vi "test TCX read (installed 71).vi"() -> ()   [LabVIEW 2011] (continued)
ts></TPX></Extensions></Trackpoint><Trackpoint><Time>2008-03-03T14:03:14Z</Time><Position><LatitudeDegrees>35.862978</LatitudeDegrees><LongitudeDegrees>-78.901660</LongitudeDegrees></Position><AltitudeMeters>94.827</AltitudeMeters><DistanceMeters>7936.581</DistanceMeters><Cadence>76</Cadence><Extensions><TPX xmlns=\"http://www.garmin.com/xmlschemas/ActivityExtension/v2\"><Watts>189</Watts></TPX></Extensions></Trackpoint><Trackpoint><Time>2008-03-03T14:03:15Z</Time><Position><LatitudeDegrees>35.862989</LatitudeDegrees><LongitudeDegrees>-78.901582</LongitudeDegrees></Position><AltitudeMeters>94.347</AltitudeMeters><DistanceMeters>7943.796</DistanceMeters><Cadence>76</Cadence><Extensions><TPX xmlns=\"http://www.garmin.com/xmlschemas/ActivityExtension/v2\"><Watts>189</Watts></TPX></Extensions></Trackpoint><Trackpoint><Time>2008-03-03T14:03:16Z</Time><Position><LatitudeDegrees>35.863009</LatitudeDegrees><LongitudeDegrees>-78.901503</LongitudeDegrees></Position><AltitudeMeters>94.347</AltitudeMeters><DistanceMeters>7951.251</DistanceMeters><Cadence>78</Cadence><Extensions><TPX xmlns=\"http://www.garmin.com/xmlschemas/ActivityExtension/v2\"><Watts>185</Watts></TPX></Extensions></Trackpoint><Trackpoint><Time>2008-03-03T14:03:17Z</Time><Position><LatitudeDegrees>35.863023</LatitudeDegrees><LongitudeDegrees>-78.901423</LongitudeDegrees></Position><AltitudeMeters>94.347</AltitudeMeters><DistanceMeters>7958.711</DistanceMeters><Cadence>78</Cadence><Extensions><TPX xmlns=\"http://www.garmin.com/xmlschemas/ActivityExtension/v2\"><Watts>184</Watts></TPX></Extensions></Trackpoint><Trackpoint><Time>2008-03-03T14:03:18Z</Time><Position><LatitudeDegrees>35.863042</LatitudeDegrees><LongitudeDegrees>-78.901342</LongitudeDegrees></Position><AltitudeMeters>94.347</AltitudeMeters><DistanceMeters>7966.281</DistanceMeters><Cadence>72</Cadence><Extensions><TPX xmlns=\"http://www.garmin.com/xmlschemas/ActivityExtension/v2\"><Watts>157</Watts></TPX></Extensions></Trackpoint><Trackpoint><Time>2008-03-03T14:03:19Z</Time><Position><LatitudeDegrees>35.863061</LatitudeDegrees><LongitudeDegrees>-78.901258</LongitudeDegrees></Position><AltitudeMeters>94.347</AltitudeMeters><DistanceMeters>7974.119</DistanceMeters><Cadence>73</Cadence><Extensions><TPX xmlns=\"http://www.garmin.com/xmlschemas/ActivityExtension/v2\"><Watts>157</Watts></TPX></Extensions></Trackpoint><Trackpoint><Time>2008-03-03T14:03:20Z</Time><Position><LatitudeDegrees>35.863074</LatitudeDegrees><LongitudeDegrees>-78.901173</LongitudeDegrees></Position><AltitudeMeters>94.347</AltitudeMeters><DistanceMeters>7981.873</DistanceMeters><Cadence>73</Cadence><Extensions><TPX xmlns=\"http://www.garmin.com/xmlschemas/ActivityExtension/v2\"><Watts>156</Watts></TPX></Extensions></Trackpoint><Trackpoint><Time>2008-03-03T14:03:21Z</Time><Position><LatitudeDegrees>35.863089</LatitudeDegrees><LongitudeDegrees>-78.901086</LongitudeDegrees></Position><AltitudeMeters>94.347</AltitudeMeters><DistanceMeters>7989.980</DistanceMeters><Cadence>78</Cadence><Extensions><TPX xmlns=\"http://www.garmin.com/xmlschemas/ActivityExtension/v2\"><Watts>181</Watts></TPX></Extensions></Trackpoint><Trackpoint><Time>2008-03-03T14:03:22Z</Time><Position><LatitudeDegrees>35.863110</LatitudeDegrees><LongitudeDegrees>-78.900992</LongitudeDegrees></Position><AltitudeMeters>93.866</AltitudeMeters><DistanceMeters>7998.730</DistanceMeters><Cadence>80</Cadence><Extensions><TPX xmlns=\"http://www.garmin.com/xmlschemas/ActivityExtension/v2\"><Watts>180</Watts></TPX></Extensions></Trackpoint><Trackpoint><Time>2008-03-03T14:03:23Z</Time><Position><LatitudeDegrees>35.863126</LatitudeDegrees><LongitudeDegrees>-78.900894</LongitudeDegrees></Position><AltitudeMeters>93.866</AltitudeMeters><DistanceMeters>8007.869</DistanceMeters><Cadence>83</Cadence><Extensions><TPX xmlns=\"http://www.garmin.com/xmlschemas/ActivityExtension/v2\"><Watts>159</Watts></TPX></Extensions></Trackpoint><Trackpoint><Time>2008-03-03T14:03:24Z</Time><Position><LatitudeDegrees>35.863147</LatitudeDegrees><LongitudeDegrees>-78.900793</LongitudeDegrees></Position><AltitudeMeters>93.866</AltitudeMeters><DistanceMeters>8017.229</DistanceMeters><Cadence>88</Cadence><Extensions><TPX xmlns=\"http://www.garmin.com/xmlschemas/ActivityExtension/v2\"><Watts>159</Watts></TPX></Extensions></Trackpoint><Trackpoint><Time>2008-03-03T14:03:25Z</Time><Position><LatitudeDegrees>35.863168</LatitudeDegrees><LongitudeDegrees>-78.900690</LongitudeDegrees></Position><AltitudeMeters>93.385</AltitudeMeters><DistanceMeters>8026.872</DistanceMeters><Cadence>88</Cadence><Extensions><TPX xmlns=\"http://www.garmin.com/xmlschemas/ActivityExtension/v2\"><Watts>159</Watts></TPX></Extensions></Trackpoint><Trackpoint><Time>2008-03-03T14:03:26Z</Time><Position><LatitudeDegrees>35.863186</LatitudeDegrees><LongitudeDegrees>-78.900583</LongitudeDegrees></Position><AltitudeMeters>92.905</AltitudeMeters><DistanceMeters>8036.698</DistanceMeters><Cadence>91</Cadence><Extensions><TPX xmlns=\"http://www.garmin.com/xmlschemas/ActivityExtension/v2\"><Watts>143</Watts></TPX></Extensions></Trackpoint><Trackpoint><Time>2008-03-03T14:03:27Z</Time><Position><LatitudeDegrees>35.863206</LatitudeDegrees><LongitudeDegrees>-78.900473</LongitudeDegrees></Position><AltitudeMeters>92.905</AltitudeMeters><DistanceMeters>8046.873</DistanceMeters><Cadence>91</Cadence><Extensions><TPX xmlns=\"http://www.garmin.com/xmlschemas/ActivityExtension/v2\"><Watts>142</Watts></TPX></Extensions></Trackpoint><Trackpoint><Time>2008-03-03T14:03:28Z</Time><Position><LatitudeDegrees>35.863225</LatitudeDegrees><LongitudeDegrees>-78.900361</LongitudeDegrees></Position><AltitudeMeters>92.424</AltitudeMeters><DistanceMeters>8057.292</DistanceMeters><Cadence>91</Cadence><Extensions><TPX xmlns=\"http://www.garmin.com/xmlschemas/ActivityExtension/v2\"><Watts>149</Watts></TPX></Extensions></Trackpoint><Trackpoint><Time>2008-03-03T14:03:29Z</Time><Position><LatitudeDegrees>35.863246</LatitudeDegrees><LongitudeDegrees>-78.900251</LongitudeDegrees></Position><AltitudeMeters>92.424</AltitudeMeters><DistanceMeters>8067.389</DistanceMeters><Cadence>91</Cadence><Extensions><TPX xmlns=\"http://www.garmin.com/xmlschemas/ActivityExtension/v2\"><Watts>148</Watts></TPX></Extensions></Trackpoint><Trackpoint><Time>2008-03-03T14:03:30Z</Time><Position><LatitudeDegrees>35.863261</LatitudeDegrees><LongitudeDegrees>-78.900148</LongitudeDegrees></Position><AltitudeMeters>92.905</AltitudeMeters><DistanceMeters>8076.814</DistanceMeters><Cadence>88</Cadence><Extensions><TPX xmlns=\"http://www.garmin.com/xmlschemas/ActivityExtension/v2\"><Watts>154</Watts></TPX></Extensions></Trackpoint><Trackpoint><Time>2008-03-03T14:03:31Z</Time><Position><LatitudeDegrees>35.863276</LatitudeDegrees><LongitudeDegrees>-78.900048</LongitudeDegrees></Position><AltitudeMeters>92.905</AltitudeMeters><DistanceMeters>8085.958</DistanceMeters><Cadence>84</Cadence><Extensions><TPX xmlns=\"http://www.garmin.com/xmlschemas/ActivityExtension/v2\"><Watts>164</Watts></TPX></Extensions></Trackpoint><Trackpoint><Time>2008-03-03T14:03:32Z</Time><Position><LatitudeDegrees>35.863288</LatitudeDegrees><LongitudeDegrees>-78.899952</LongitudeDegrees></Position><AltitudeMeters>92.905</AltitudeMeters><DistanceMeters>8094.699</DistanceMeters><Cadence>83</Cadence><Extensions><TPX xmlns=\"http://www.garmin.com/xmlschemas/ActivityExtension/v2\"><Watts>165</Watts></TPX></Extensions></Trackpoint><Trackpoint><Time>2008-03-03T14:03:33Z</Time><Position><LatitudeDegrees>35.863300</LatitudeDegrees><LongitudeDegrees>-78.899857</LongitudeDegrees></Position><AltitudeMeters>93.385</AltitudeMeters><DistanceMeters>8103.383</DistanceMeters><Cadence>79</Cadence><Extensions><TPX xmlns=\"http://www.garmin.com/xmlschemas/ActivityExtension/v2\"><Watts>173</Watts></TPX></Extensions></Trackpoint><Trackpoint><Time>2008-03-03T14:03:34Z</Time><Position><LatitudeDegrees>35.863310</LatitudeDegrees><LongitudeDegrees>-78.899768</LongitudeDegrees></Position><AltitudeMeters>93.385</AltitudeMeters><DistanceMeters>8111.526</DistanceMeters><Cadence>74</Cadence><Extensions><TPX xmlns=\"http://www.garmin.com/xmlschemas/ActivityExtension/v2\"><Watts>185</Watts></TPX></Extensions></Trackpoint><Trackpoint><Time>2008-03-03T14:03:35Z</Time><Position><LatitudeDegrees>35.863325</LatitudeDegrees><LongitudeDegrees>-78.899681</LongitudeDegrees></Position><AltitudeMeters>93.866</AltitudeMeters><DistanceMeters>8119.541</DistanceMeters><Cadence>74</Cadence><Extensions><TPX xmlns=\"http://www.garmin.com/xmlschemas/ActivityExtension/v2\"><Watts>186</Watts></TPX></Extensions></Trackpoint><Trackpoint><Time>2008-03-03T14:03:36Z</Time><Position><LatitudeDegrees>35.863345</LatitudeDegrees><LongitudeDegrees>-78.899593</LongitudeDegrees></Position><AltitudeMeters>93.866</AltitudeMeters><DistanceMeters>8127.668</DistanceMeters><Cadence>75</Cadence><Extensions><TPX xmlns=\"http://www.garmin.com/xmlschemas/ActivityExtension/v2\"><Watts>416</Watts></TPX></Extensions></Trackpoint><Trackpoint><Time>2008-03-03T14:03:37Z</Time><Position><LatitudeDegrees>35.863368</LatitudeDegrees><LongitudeDegrees>-78.899510</LongitudeDegrees></Position><AltitudeMeters>94.827</AltitudeMeters><DistanceMeters>8135.531</DistanceMeters><Cadence>75</Cadence><Extensions><TPX xmlns=\"http://www.garmin.com/xmlschemas/ActivityExtension/v2\"><Watts>415</Watts></TPX></Extensions></Trackpoint><Trackpoint><Time>2008-03-03T14:03:38Z</Time><Position><LatitudeDegrees>35.863381</LatitudeDegrees><LongitudeDegrees>-78.899422</LongitudeDegrees></Position><AltitudeMeters>94.827</AltitudeMeters><DistanceMeters>8143.633</DistanceMeters><Cadence>77</Cadence><Extensions><TPX xmlns=\"http://www.garmin.com/xmlschemas/ActivityExtension/v2\"><Watts>685</Watts></TPX></Extensions></Trackpoint><Trackpoint><Time>2008-03-03T14:03:39Z</Time><Position><LatitudeDegrees>35.863397</LatitudeDegrees><LongitudeDegrees>-78.899329</LongitudeDegrees></Position><AltitudeMeters>95.308</AltitudeMeters><DistanceMeters>8152.224</DistanceMeters><Cadence>78</Cadence><Extensions><TPX xmlns=\"http://www.garmin.com/xmlschemas/ActivityExtension/v2\"><Watts>675</Watts></TPX></Extensions></Trackpoint><Trackpoint><Time>2008-03-03T14:03:40Z</Time><Position><LatitudeDegrees>35.863421</LatitudeDegrees><LongitudeDegrees>-78.899235</LongitudeDegrees></Position><AltitudeMeters>95.788</AltitudeMeters><DistanceMeters>8161.086</DistanceMeters><Cadence>79</Cadence><Extensions><TPX xmlns=\"http://www.garmin.com/xmlschemas/ActivityExtension/v2\"><Watts>674</Watts></TPX></Extensions></Trackpoint><Trackpoint><Time>2008-03-03T14:03:41Z</Time><Position><LatitudeDegrees>35.863439</LatitudeDegrees><LongitudeDegrees>-78.899142</LongitudeDegrees></Position><AltitudeMeters>96.269</AltitudeMeters><DistanceMeters>8169.801</DistanceMeters><Cadence>79</Cadence><Extensions><TPX xmlns=\"http://www.garmin.com/xmlschemas/ActivityExtension/v2\"><Watts>667</Watts></TPX></Extensions></Trackpoint><Trackpoint><Time>2008-03-03T14:03:42Z</Time><Position><LatitudeDegrees>35.863455</LatitudeDegrees><LongitudeDegrees>-78.899045</LongitudeDegrees></Position><AltitudeMeters>96.269</AltitudeMeters><DistanceMeters>8178.699</DistanceMeters><Cadence>79</Cadence><Extensions><TPX xmlns=\"http://www.garmin.com/xmlschemas/ActivityExtension/v2\"><Watts>670</Watts></TPX></Extensions></Trackpoint><Trackpoint><Time>2008-03-03T14:03:43Z</Time><Position><LatitudeDegrees>35.863473</LatitudeDegrees><LongitudeDegrees>-78.898952</LongitudeDegrees></Position><AltitudeMeters>96.750</AltitudeMeters><DistanceMeters>8187.334</DistanceMeters><Cadence>79</Cadence><Extensions><TPX xmlns=\"http://www.garmin.com/xmlschemas/ActivityExtension/v2\"><Watts>540</Watts></TPX></Extensions></Trackpoint><Trackpoint><Time>2008-03-03T14:03:44Z</Time><Position><LatitudeDegrees>35.863492</LatitudeDegrees><LongitudeDegrees>-78.898856</LongitudeDegrees></Position><AltitudeMeters>96.750</AltitudeMeters><DistanceMeters>8196.224</DistanceMeters><Cadence>79</Cadence><Extensions><TPX xmlns=\"http://www.garmin.com/xmlschemas/ActivityExtension/v2\"><Watts>544</Watts></TPX></Extensions></Trackpoint><Trackpoint><Time>2008-03-03T14:03:45Z</Time><Position><LatitudeDegrees>35.863502</LatitudeDegrees><LongitudeDegrees>-78.898763</LongitudeDegrees></Position><AltitudeMeters>97.711</AltitudeMeters><DistanceMeters>8204.663</DistanceMeters><Cadence>79</Cadence><Extensions><TPX xmlns=\"http://www.garmin.com/xmlschemas/ActivityExtension/v2\"><Watts>541</Watts></TPX></Extensions></Trackpoint><Trackpoint><Time>2008-03-03T14:03:46Z</Time><Position><LatitudeDegrees>35.863514</LatitudeDegrees><LongitudeDegrees>-78.898672</LongitudeDegrees></Position><AltitudeMeters>97.711</AltitudeMeters><DistanceMeters>8212.996</DistanceMeters><Cadence>78</Cadence><Extensions><TPX xmlns=\"http://www.garmin.com/xmlschemas/ActivityExtension/v2\"><Watts>515</Watts></TPX></Extensions></Trackpoint><Trackpoint><Time>2008-03-03T14:03:47Z</Time><Position><LatitudeDegrees>35.863528</LatitudeDegrees><LongitudeDegrees>-78.898578</LongitudeDegrees></Position><AltitudeMeters>98.192</AltitudeMeters><DistanceMeters>8221.674</DistanceMeters><Cadence>79</Cadence><Extensions><TPX xmlns=\"http://www.garmin.com/xmlschemas/ActivityExtension/v2\"><Watts>507</Watts></TPX></Extensions></Trackpoint><Trackpoint><Time>2008-03-03T14:03:48Z</Time><Position><LatitudeDegrees>35.863539</LatitudeDegrees><LongitudeDegrees>-78.898486</LongitudeDegrees></Position><AltitudeMeters>98.192</AltitudeMeters><DistanceMeters>8230.088</DistanceMeters><Cadence>79</Cadence><Extensions><TPX xmlns=\"http://www.garmin.com/xmlschemas/ActivityExtension/v2\"><Watts>482</Watts></TPX></Extensions></Trackpoint><Trackpoint><Time>2008-03-03T14:03:49Z</Time><Position><LatitudeDegrees>35.863548</LatitudeDegrees><LongitudeDegrees>-78.898391</LongitudeDegrees></Position><AltitudeMeters>99.153</AltitudeMeters><DistanceMeters>8238.679</DistanceMeters><Cadence>81</Cadence><Extensions><TPX xmlns=\"http://www.garmin.com/xmlschemas/ActivityExtension/v2\"><Watts>470</Watts></TPX></Extensions></Trackpoint><Trackpoint><Time>2008-03-03T14:03:50Z</Time><Position><LatitudeDegrees>35.863565</LatitudeDegrees><LongitudeDegrees>-78.898296</LongitudeDegrees></Position><AltitudeMeters>99.153</AltitudeMeters><DistanceMeters>8247.451</DistanceMeters><Cadence>78</Cadence><Extensions><TPX xmlns=\"http://www.garmin.com/xmlschemas/ActivityExtension/v2\"><Watts>381</Watts></TPX></Extensions></Trackpoint><Trackpoint><Time>2008-03-03T14:03:51Z</Time><Position><LatitudeDegrees>35.863576</LatitudeDegrees><LongitudeDegrees>-78.898206</LongitudeDegrees></Position><AltitudeMeters>99.634</AltitudeMeters><DistanceMeters>8255.699</DistanceMeters><Cadence>77</Cadence><Extensions><TPX xmlns=\"http://www.garmin.com/xmlschemas/ActivityExtension/v2\"><Watts>278</Watts></TPX></Extensions></Trackpoint><Trackpoint><Time>2008-03-03T14:03:52Z</Time><Position><LatitudeDegrees>35.863592</LatitudeDegrees><LongitudeDegrees>-78.898116</LongitudeDegrees></Position><AltitudeMeters>99.634</AltitudeMeters><DistanceMeters>8264.034</DistanceMeters><Cadence>77</Cadence><Extensions><TPX xmlns=\"http://www.garmin.com/xmlschemas/ActivityExtension/v2\"><Watts>278</Watts></TPX></Extensions></Trackpoint><Trackpoint><Time>2008-03-03T14:03:53Z</Time><Position><LatitudeDegrees>35.863607</LatitudeDegrees><LongitudeDegrees>-78.898024</LongitudeDegrees></Position><AltitudeMeters>100.115</AltitudeMeters><DistanceMeters>8272.420</DistanceMeters><Cadence>75</Cadence><Extensions><TPX xmlns=\"http://www.garmin.com/xmlschemas/ActivityExtension/v2\"><Watts>223</Watts></TPX></Extensions></Trackpoint><Trackpoint><Time>2008-03-03T14:03:54Z</Time><Position><LatitudeDegrees>35.863619</LatitudeDegrees><LongitudeDegrees>-78.897934</LongitudeDegrees></Position><AltitudeMeters>100.115</AltitudeMeters><DistanceMeters>8280.670</DistanceMeters><Cadence>75</Cadence><Extensions><TPX xmlns=\"http://www.garmin.com/xmlschemas/ActivityExtension/v2\"><Watts>222</Watts></TPX></Extensions></Trackpoint><Trackpoint><Time>2008-03-03T14:03:55Z</Time><Position><LatitudeDegrees>35.863635</LatitudeDegrees><LongitudeDegrees>-78.897846</LongitudeDegrees></Position><AltitudeMeters>100.115</AltitudeMeters><DistanceMeters>8288.826</DistanceMeters><Cadence>73</Cadence><Extensions><TPX xmlns=\"http://www.garmin.com/xmlschemas/ActivityExtension/v2\"><Watts>224</Watts></TPX></Extensions></Trackpoint><Trackpoint><Time>2008-03-03T14:03:56Z</Time><Position><LatitudeDegrees>35.863646</LatitudeDegrees><LongitudeDegrees>-78.897761</LongitudeDegrees></Position><AltitudeMeters>100.115</AltitudeMeters><DistanceMeters>8296.627</DistanceMeters><Cadence>73</Cadence><Extensions><TPX xmlns=\"http://www.garmin.com/xmlschemas/ActivityExtension/v2\"><Watts>224</Watts></TPX></Extensions></Trackpoint><Trackpoint><Time>2008-03-03T14:03:57Z</Time><Position><LatitudeDegrees>35.863663</LatitudeDegrees><LongitudeDegrees>-78.897678</LongitudeDegrees></Position><AltitudeMeters>100.595</AltitudeMeters><DistanceMeters>8304.372</DistanceMeters><Cadence>72</Cadence><Extensions><TPX xmlns=\"http://www.garmin.com/xmlschemas/ActivityExtension/v2\"><Watts>221</Watts></TPX></Extensions></Trackpoint><Trackpoint><Time>2008-03-03T14:03:58Z</Time><Position><LatitudeDegrees>35.863680</LatitudeDegrees><LongitudeDegrees>-78.897595</LongitudeDegrees></Position><AltitudeMeters>100.595</AltitudeMeters><DistanceMeters>8312.060</DistanceMeters><Cadence>70</Cadence><Extensions><TPX xmlns=\"http://www.garmin.com/xmlschemas/ActivityExtension/v2\"><Watts>207</Watts></TPX></Extensions></Trackpoint><Trackpoint><Time>2008-03-03T14:03:59Z</Time><Position><LatitudeDegrees>35.863703</LatitudeDegrees><LongitudeDegrees>-78.897514</LongitudeDegrees></Position><AltitudeMeters>101.076</AltitudeMeters><DistanceMeters>8319.789</DistanceMeters><Cadence>69</Cadence><Extensions><TPX xmlns=\"http://www.garmin.com/xmlschemas/ActivityExtension/v2\"><Watts>193</Watts></TPX></Extensions></Trackpoint><Trackpoint><Time>2008-03-03T14:04:00Z</Time><Position><LatitudeDegrees>35.863717</LatitudeDegrees><LongitudeDegrees>-78.897436</LongitudeDegrees></Position><AltitudeMeters>101.076</AltitudeMeters><DistanceMeters>8327.021</DistanceMeters><Cadence>67</Cadence><Extensions><TPX xmlns=\"http://www.garmin.com/xmlschemas/ActivityExtension/v2\"><Watts>198</Watts></TPX></Extensions></Trackpoint><Trackpoint><Time>2008-03-03T14:04:01Z</Time><Position><LatitudeDegrees>35.863723</LatitudeDegrees><LongitudeDegrees>-78.897357</LongitudeDegrees></Position><AltitudeMeters>101.076</AltitudeMeters><DistanceMeters>8334.132</DistanceMeters><Cadence>67</Cadence><Extensions><TPX xmlns=\"http://www.garmin.com/xmlschemas/ActivityExtension/v2\"><Watts>215</Watts></TPX></Extensions></Trackpoint><Trackpoint><Time>2008-03-03T14:04:02Z</Time><Position><LatitudeDegrees>35.863730</LatitudeDegrees><LongitudeDegrees>-78.897280</LongitudeDegrees></Position><AltitudeMeters>101.076</AltitudeMeters><DistanceMeters>8341.184</DistanceMeters><Cadence>67</Cadence><Extensions><TPX xmlns=\"http://www.garmin.com/xmlschemas/ActivityExtension/v2\"><Watts>213</Watts></TPX></Extensions></Trackpoint><Trackpoint><Time>2008-03-03T14:04:03Z</Time><Position><LatitudeDegrees>35.863739</LatitudeDegrees><LongitudeDegrees>-78.897199</LongitudeDegrees></Position><AltitudeMeters>101.076</AltitudeMeters><DistanceMeters>8348.546</DistanceMeters><Cadence>67</Cadence><Extensions><TPX xmlns=\"http://www.garmin.com/xmlschemas/ActivityExtension/v2\"><Watts>230</Watts></TPX></Extensions></Trackpoint><Trackpoint><Time>2008-03-03T14:04:04Z</Time><Position><LatitudeDegrees>35.863747</LatitudeDegrees><LongitudeDegrees>-78.897118</LongitudeDegrees></Position><AltitudeMeters>101.076</AltitudeMeters><DistanceMeters>8355.904</DistanceMeters><Cadence>67</Cadence><Extensions><TPX xmlns=\"http://www.garmin.com/xmlschemas/ActivityExtension/v2\"><Watts>232</Watts></TPX></Extensions></Trackpoint><Trackpoint><Time>2008-03-03T14:04:05Z</Time><Position><LatitudeDegrees>35.863738</LatitudeDegrees><LongitudeDegrees>-78.897041</LongitudeDegrees></Position><AltitudeMeters>101.076</AltitudeMeters><DistanceMeters>8362.927</DistanceMeters><Cadence>66</Cadence><Extensions><TPX xmlns=\"http://www.garmin.com/xmlschemas/ActivityExtension/v2\"><Watts>158</Watts></TPX></Extensions></Trackpoint><Trackpoint><Time>2008-03-03T14:04:06Z</Time><Position><LatitudeDegrees>35.863710</LatitudeDegrees><LongitudeDegrees>-78.896976</LongitudeDegrees></Position><AltitudeMeters>101.556</AltitudeMeters><DistanceMeters>8369.553</DistanceMeters><Cadence>66</Cadence><Extensions><TPX xmlns=\"http://www.garmin.com/xmlschemas/ActivityExtension/v2\"><Watts>141</Watts></TPX></Extensions></Trackpoint><Trackpoint><Time>2008-03-03T14:04:07Z</Time><Position><LatitudeDegrees>35.863647</LatitudeDegrees><LongitudeDegrees>-78.896943</LongitudeDegrees></Position><AltitudeMeters>101.556</AltitudeMeters><DistanceMeters>8377.287</DistanceMeters><Cadence>66</Cadence><Extensions><TPX xmlns=\"http://www.garmin.com/xmlschemas/ActivityExtension/v2\"><Watts>141</Watts></TPX></Extensions></Trackpoint><Trackpoint><Time>2008-03-03T14:04:08Z</Time><Position><LatitudeDegrees>35.863588</LatitudeDegrees><LongitudeDegrees>-78.896935</LongitudeDegrees></Position><AltitudeMeters>101.556</AltitudeMeters><DistanceMeters>8383.846</DistanceMeters><Cadence>66</Cadence><Extensions><TPX xmlns=\"http://www.garmin.com/xmlschemas/ActivityExtension/v2\"><Watts>136</Watts></TPX></Extensions></Trackpoint><Trackpoint><Time>2008-03-03T14:04:09Z</Time><Position><LatitudeDegrees>35.863528</LatitudeDegrees><LongitudeDegrees>-78.896946</LongitudeDegrees></Position><AltitudeMeters>101.556</AltitudeMeters><DistanceMeters>8390.634</DistanceMeters><Cadence>66</Cadence><Extensions><TPX xmlns=\"http://www.garmin.com/xmlschemas/ActivityExtension/v2\"><Watts>135</Watts></TPX></Extensions></Trackpoint><Trackpoint><Time>2008-03-03T14:04:10Z</Time><Position><LatitudeDegrees>35.863467</LatitudeDegrees><LongitudeDegrees>-78.896965</LongitudeDegrees></Position><AltitudeMeters>101.556</AltitudeMeters><DistanceMeters>8397.591</DistanceMeters><Cadence>67</Cadence><Extensions><TPX xmlns=\"http://www.garmin.com/xmlschemas/ActivityExtension/v2\"><Watts>130</Watts></TPX></Extensions></Trackpoint><Trackpoint><Time>2008-03-03T14:04:11Z</Time><Position><LatitudeDegrees>35.863399</LatitudeDegrees><LongitudeDegrees>-78.896982</LongitudeDegrees></Position><AltitudeMeters>101.556</AltitudeMeters><DistanceMeters>8405.279</DistanceMeters><Cadence>67</Cadence><Extensions><TPX xmlns=\"http://www.garmin.com/xmlschemas/ActivityExtension/v2\"><Watts>141</Watts></TPX></Extensions></Trackpoint><Trackpoint><Time>2008-03-03T14:04:12Z</Time><Position><LatitudeDegrees>35.863331</LatitudeDegrees><LongitudeDegrees>-78.896996</LongitudeDegrees></Position><AltitudeMeters>101.556</AltitudeMeters><DistanceMeters>8412.914</DistanceMeters><Cadence>68</Cadence><Extensions><TPX xmlns=\"http://www.garmin.com/xmlschemas/ActivityExtension/v2\"><Watts>151</Watts></TPX></Extensions></Trackpoint><Trackpoint><Time>2008-03-03T14:04:13Z</Time><Position><LatitudeDegrees>35.863263</LatitudeDegrees><LongitudeDegrees>-78.897010</LongitudeDegrees></Position><AltitudeMeters>101.556</AltitudeMeters><DistanceMeters>8420.536</DistanceMeters><Cadence>70</Cadence><Extensions><TPX xmlns=\"http://www.garmin.com/xmlschemas/ActivityExtension/v2\"><Watts>158</Watts></TPX></Extensions></Trackpoint><Trackpoint><Time>2008-03-03T14:04:14Z</Time><Position><LatitudeDegrees>35.863190</LatitudeDegrees><LongitudeDegrees>-78.897026</LongitudeDegrees></Position><AltitudeMeters>102.037</AltitudeMeters><DistanceMeters>8428.863</DistanceMeters><Cadence>71</Cadence><Extensions><TPX xmlns=\"http://www.garmin.com/xmlschemas/ActivityExtension/v2\"><Watts>158</Watts></TPX></Extensions></Trackpoint><Trackpoint><Time>2008-03-03T14:04:15Z</Time><Position><LatitudeDegrees>35.863116</LatitudeDegrees><LongitudeDegrees>-78.897046</LongitudeDegrees></Position><AltitudeMeters>102.037</AltitudeMeters><DistanceMeters>8437.228</DistanceMeters><Cadence>72</Cadence><Extensions><TPX xmlns=\"http://www.garmin.com/xmlschemas/ActivityExtension/v2\"><Watts>132</Watts></TPX></Extensions></Trackpoint><Trackpoint><Time>2008-03-03T14:04:16Z</Time><Position><LatitudeDegrees>35.863041</LatitudeDegrees><LongitudeDegrees>-78.897060</LongitudeDegrees></Position><AltitudeMeters>102.037</AltitudeMeters><DistanceMeters>8445.677</DistanceMeters><Cadence>73</Cadence><Extensions><TPX xmlns=\"http://www.garmin.com/xmlschemas/ActivityExtension/v2\"><Watts>127</Watts></TPX></Extensions></Trackpoint><Trackpoint><Time>2008-03-03T14:04:17Z</Time><Position><LatitudeDegrees>35.862967</LatitudeDegrees><LongitudeDegrees>-78.897071</LongitudeDegrees></Position><AltitudeMeters>102.037</AltitudeMeters><DistanceMeters>8453.937</DistanceMeters><Cadence>73</Cadence><Extensions><TPX xmlns=\"http://www.garmin.com/xmlschemas/ActivityExtension/v2\"><Watts>127</Watts></TPX></Extensions></Trackpoint><Trackpoint><Time>2008-03-03T14:04:18Z</Time><Position><LatitudeDegrees>35.862899</LatitudeDegrees><LongitudeDegrees>-78.897083</LongitudeDegrees></Position><AltitudeMeters>102.037</AltitudeMeters><DistanceMeters>8461.561</DistanceMeters><Cadence>73</Cadence><Extensions><TPX xmlns=\"http://www.garmin.com/xmlschemas/ActivityExtension/v2\"><Watts>119</Watts></TPX></Extensions></Trackpoint><Trackpoint><Time>2008-03-03T14:04:19Z</Time><Position><LatitudeDegrees>35.862828</LatitudeDegrees><LongitudeDegrees>-78.897094</LongitudeDegrees></Position><AltitudeMeters>101.556</AltitudeMeters><DistanceMeters>8469.438</DistanceMeters><Cadence>73</Cadence><Extensions><TPX xmlns=\"http://www.garmin.com/xmlschemas/ActivityExtension/v2\"><Watts>120</Watts></TPX></Extensions></Trackpoint><Trackpoint><Time>2008-03-03T14:04:20Z</Time><Position><LatitudeDegrees>35.862757</LatitudeDegrees><LongitudeDegrees>-78.897104</LongitudeDegrees></Position><AltitudeMeters>101.076</AltitudeMeters><DistanceMeters>8477.459</DistanceMeters><Cadence>75</Cadence><Extensions><TPX xmlns=\"http://www.garmin.com/xmlschemas/ActivityExtension/v2\"><Watts>129</Watts></TPX></Extensions></Trackpoint><Trackpoint><Time>2008-03-03T14:04:21Z</Time><Position><LatitudeDegrees>35.862683</LatitudeDegrees><LongitudeDegrees>-78.897116</LongitudeDegrees></Position><AltitudeMeters>101.076</AltitudeMeters><DistanceMeters>8485.744</DistanceMeters><Cadence>76</Cadence><Extensions><TPX xmlns=\"http://www.garmin.com/xmlschemas/ActivityExtension/v2\"><Watts>129</Watts></TPX></Extensions></Trackpoint><Trackpoint><Time>2008-03-03T14:04:22Z</Time><Position><LatitudeDegrees>35.862610</LatitudeDegrees><LongitudeDegrees>-78.897129</LongitudeDegrees></Position><AltitudeMeters>101.076</AltitudeMeters><DistanceMeters>8493.926</DistanceMeters><Cadence>77</Cadence><Extensions><TPX xmlns=\"http://www.garmin.com/xmlschemas/ActivityExtension/v2\"><Watts>129</Watts></TPX></Extensions></Trackpoint><Trackpoint><Time>2008-03-03T14:04:23Z</Time><Position><LatitudeDegrees>35.862534</LatitudeDegrees><LongitudeDegrees>-78.897142</LongitudeDegrees></Position><AltitudeMeters>100.115</AltitudeMeters><DistanceMeters>8502.362</DistanceMeters><Cadence>78</Cadence><Extensions><TPX xmlns=\"http://www.garmin.com/xmlschemas/ActivityExtension/v2\"><Watts>116</Watts></TPX></Extensions></Trackpoint><Trackpoint><Time>2008-03-03T14:04:24Z</Time><Position><LatitudeDegrees>35.862457</LatitudeDegrees><LongitudeDegrees>-78.897159</LongitudeDegrees></Position><AltitudeMeters>100.115</AltitudeMeters><DistanceMeters>8511.070</DistanceMeters><Cadence>78</Cadence><Extensions><TPX xmlns=\"http://www.garmin.com/xmlschemas/ActivityExtension/v2\"><Watts>116</Watts></TPX></Extensions></Trackpoint><Trackpoint><Time>2008-03-03T14:04:25Z</Time><Position><LatitudeDegrees>35.862384</LatitudeDegrees><LongitudeDegrees>-78.897181</LongitudeDegrees></Position><AltitudeMeters>99.634</AltitudeMeters><DistanceMeters>8519.451</DistanceMeters><Cadence>78</Cadence><Extensions><TPX xmlns=\"http://www.garmin.com/xmlschemas/ActivityExtension/v2\"><Watts>110</Watts></TPX></Extensions></Trackpoint><Trackpoint><Time>2008-03-03T14:04:26Z</Time><Position><LatitudeDegrees>35.862311</LatitudeDegrees><LongitudeDegrees>-78.897205</LongitudeDegrees></Position><AltitudeMeters>99.153</AltitudeMeters><DistanceMeters>8527.767</DistanceMeters><Cadence>78</Cadence><Extensions><TPX xmlns=\"http://www.garmin.com/xmlschemas/ActivityExtension/v2\"><Watts>108</Watts></TPX></Extensions></Trackpoint><Trackpoint><Time>2008-03-03T14:04:27Z</Time><Position><LatitudeDegrees>35.862235</LatitudeDegrees><LongitudeDegrees>-78.897229</LongitudeDegrees></Position><AltitudeMeters>98.672</AltitudeMeters><DistanceMeters>8536.483</DistanceMeters><Cadence>80</Cadence><Extensions><TPX xmlns=\"http://www.garmin.com/xmlschemas/ActivityExtension/v2\"><Watts>104</Watts></TPX></Extensions></Trackpoint><Trackpoint><Time>2008-03-03T14:04:28Z</Time><Position><LatitudeDegrees>35.862161</LatitudeDegrees><LongitudeDegrees>-78.897257</LongitudeDegrees></Position><AltitudeMeters>99.153</AltitudeMeters><DistanceMeters>8545.181</DistanceMeters><Cadence>81</Cadence><Extensions><TPX xmlns=\"http://www.garmin.com/xmlschemas/ActivityExtension/v2\"><Watts>101</Watts></TPX></Extensions></Trackpoint><Trackpoint><Time>2008-03-03T14:04:29Z</Time><Position><LatitudeDegrees>35.862088</LatitudeDegrees><LongitudeDegrees>-78.897289</LongitudeDegrees></Position><AltitudeMeters>98.672</AltitudeMeters><DistanceMeters>8553.725</DistanceMeters><Cadence>81</Cadence><Extensions><TPX xmlns=\"http://www.garmin.com/xmlschemas/ActivityExtension/v2\"><Watts>102</Watts></TPX></Extensions></Trackpoint><Trackpoint><Time>2008-03-03T14:04:30Z</Time><Position><LatitudeDegrees>35.862015</LatitudeDegrees><LongitudeDegrees>-78.897322</LongitudeDegrees></Position><AltitudeMeters>99.153</AltitudeMeters><DistanceMeters>8562.310</DistanceMeters><Cadence>72</Cadence><Extensions><TPX xmlns=\"http://www.garmin.com/xmlschemas/ActivityExtension/v2\"><Watts>99</Watts></TPX></Extensions></Trackpoint><Trackpoint><Time>2008-03-03T14:04:31Z</Time><Position><LatitudeDegrees>35.861941</LatitudeDegrees><LongitudeDegrees>-78.897358</LongitudeDegrees></Position><AltitudeMeters>98.672</AltitudeMeters><DistanceMeters>8571.180</DistanceMeters><Cadence>72</Cadence><Extensions><TPX xmlns=\"http://www.garmin.com/xmlschemas/ActivityExtension/v2\"><Watts>99</Watts></TPX></Extensions></Trackpoint><Trackpoint><Time>2008-03-03T14:04:32Z</Time><Position><LatitudeDegrees>35.861868</LatitudeDegrees><LongitudeDegrees>-78.897396</LongitudeDegrees></Position><AltitudeMeters>98.672</AltitudeMeters><DistanceMeters>8580.018</DistanceMeters><Cadence>74</Cadence><Extensions><TPX xmlns=\"http://www.garmin.com/xmlschemas/ActivityExtension/v2\"><Watts>117</Watts></TPX></Extensions></Trackpoint><Trackpoint><Time>2008-03-03T14:04:33Z</Time><Position><LatitudeDegrees>35.861793</LatitudeDegrees><LongitudeDegrees>-78.897438</LongitudeDegrees></Position><AltitudeMeters>98.672</AltitudeMeters><DistanceMeters>8589.159</DistanceMeters><Cadence>75</Cadence><Extensions><TPX xmlns=\"http://www.garmin.com/xmlschemas/ActivityExtension/v2\"><Watts>146</Watts></TPX></Extensions></Trackpoint><Trackpoint><Time>2008-03-03T14:04:34Z</Time><Position><LatitudeDegrees>35.861715</LatitudeDegrees><LongitudeDegrees>-78.897481</LongitudeDegrees></Position><AltitudeMeters>98.192</AltitudeMeters><DistanceMeters>8598.698</DistanceMeters><Cadence>76</Cadence><Extensions><TPX xmlns=\"http://www.garmin.com/xmlschemas/ActivityExtension/v2\"><Watts>146</Watts></TPX></Extensions></Trackpoint><Trackpoint><Time>2008-03-03T14:04:35Z</Time><Position><LatitudeDegrees>35.861637</LatitudeDegrees><LongitudeDegrees>-78.897527</LongitudeDegrees></Position><AltitudeMeters>98.192</AltitudeMeters><DistanceMeters>8608.271</DistanceMeters><Cadence>76</Cadence><Extensions><TPX xmlns=\"http://www.garmin.com/xmlschemas/ActivityExtension/v2\"><Watts>144</Watts></TPX></Extensions></Trackpoint><Trackpoint><Time>2008-03-03T14:04:36Z</Time><Position><LatitudeDegrees>35.861561</LatitudeDegrees><LongitudeDegrees>-78.897573</LongitudeDegrees></Position><AltitudeMeters>97.230</AltitudeMeters><DistanceMeters>8617.701</DistanceMeters><Cadence>77</Cadence><Extensions><TPX xmlns=\"http://www.garmin.com/xmlschemas/ActivityExtension/v2\"><Watts>143</Watts></TPX></Extensions></Trackpoint><Trackpoint><Time>2008-03-03T14:04:37Z</Time><Position><LatitudeDegrees>35.861484</LatitudeDegrees><LongitudeDegrees>-78.897620</LongitudeDegrees></Position><AltitudeMeters>97.230</AltitudeMeters><DistanceMeters>8627.146</DistanceMeters><Cadence>77</Cadence><Extensions><TPX xmlns=\"http://www.garmin.com/xmlschemas/ActivityExtension/v2\"><Watts>162</Watts></TPX></Extensions></Trackpoint><Trackpoint><Time>2008-03-03T14:04:38Z</Time><Position><LatitudeDegrees>35.861406</LatitudeDegrees><LongitudeDegrees>-78.897660</LongitudeDegrees></Position><AltitudeMeters>97.230</AltitudeMeters><DistanceMeters>8636.559</DistanceMeters><Cadence>78</Cadence><Extensions><TPX xmlns=\"http://www.garmin.com/xmlschemas/ActivityExtension/v2\"><Watts>162</Watts></TPX></Extensions></Trackpoint><Trackpoint><Time>2008-03-03T14:04:39Z</Time><Position><LatitudeDegrees>35.861322</LatitudeDegrees><LongitudeDegrees>-78.897687</LongitudeDegrees></Position><AltitudeMeters>96.750</AltitudeMeters><DistanceMeters>8646.126</DistanceMeters><Cadence>78</Cadence><Extensions><TPX xmlns=\"http://www.garmin.com/xmlschemas/ActivityExtension/v2\"><Watts>163</Watts></TPX></Extensions></Trackpoint><Trackpoint><Time>2008-03-03T14:04:40Z</Time><Position><LatitudeDegrees>35.861236</LatitudeDegrees><LongitudeDegrees>-78.897689</LongitudeDegrees></Position><AltitudeMeters>96.269</AltitudeMeters><DistanceMeters>8655.636</DistanceMeters><Cadence>79</Cadence><Extensions><TPX xmlns=\"http://www.garmin.com/xmlschemas/ActivityExtension/v2\"><Watts>115</Watts></TPX></Extensions></Trackpoint><Trackpoint><Time>2008-03-03T14:04:41Z</Time><Position><LatitudeDegrees>35.861142</LatitudeDegrees><LongitudeDegrees>-78.897635</LongitudeDegrees></Position><AltitudeMeters>95.788</AltitudeMeters><DistanceMeters>8667.022</DistanceMeters><Cadence>79</Cadence><Extensions><TPX xmlns=\"http://www.garmin.com/xmlschemas/ActivityExtension/v2\"><Watts>116</Watts></TPX></Extensions></Trackpoint><Trackpoint><Time>2008-03-03T14:04:42Z</Time><Position><LatitudeDegrees>35.861077</LatitudeDegrees><LongitudeDegrees>-78.897553</LongitudeDegrees></Position><AltitudeMeters>95.308</AltitudeMeters><DistanceMeters>8677.458</DistanceMeters><Cadence>28</Cadence><Extensions><TPX xmlns=\"http://www.garmin.com/xmlschemas/ActivityExtension/v2\"><Watts>98</Watts></TPX></Extensions></Trackpoint><Trackpoint><Time>2008-03-03T14:04:43Z</Time><Position><LatitudeDegrees>35.861053</LatitudeDegrees><LongitudeDegrees>-78.897445</LongitudeDegrees></Position><AltitudeMeters>95.308</AltitudeMeters><DistanceMeters>8687.614</DistanceMeters><Cadence>80</Cadence><Extensions><TPX xmlns=\"http://www.garmin.com/xmlschemas/ActivityExtension/v2\"><Watts>93</Watts></TPX></Extensions></Trackpoint><Trackpoint><Time>2008-03-03T14:04:44Z</Time><Position><LatitudeDegrees>35.861034</LatitudeDegrees><LongitudeDegrees>-78.897331</LongitudeDegrees></Position><AltitudeMeters>95.308</AltitudeMeters><DistanceMeters>8698.135</DistanceMeters><Cadence>75</Cadence><Extensions><TPX xmlns=\"http://www.garmin.com/xmlschemas/ActivityExtension/v2\"><Watts>132</Watts></TPX></Extensions></Trackpoint><Trackpoint><Time>2008-03-03T14:04:45Z</Time><Position><LatitudeDegrees>35.861015</LatitudeDegrees><LongitudeDegrees>-78.897215</LongitudeDegrees></Position><AltitudeMeters>95.308</AltitudeMeters><DistanceMeters>8708.733</DistanceMeters><Cadence>76</Cadence><Extensions><TPX xmlns=\"http://www.garmin.com/xmlschemas/ActivityExtension/v2\"><Watts>160</Watts></TPX></Extensions></Trackpoint><Trackpoint><Time>2008-03-03T14:04:46Z</Time><Position><LatitudeDegrees>35.861010</LatitudeDegrees><LongitudeDegrees>-78.897101</LongitudeDegrees></Position><AltitudeMeters>94.827</AltitudeMeters><DistanceMeters>8719.034</DistanceMeters><Cadence>77</Cadence><Extensions><TPX xmlns=\"http://www.garmin.com/xmlschemas/ActivityExtension/v2\"><Watts>168</Watts></TPX></Extensions></Trackpoint><Trackpoint><Time>2008-03-03T14:04:47Z</Time><Position><LatitudeDegrees>35.861014</LatitudeDegrees><LongitudeDegrees>-78.896994</LongitudeDegrees></Position><AltitudeMeters>94.827</AltitudeMeters><DistanceMeters>8728.649</DistanceMeters><Cadence>78</Cadence><Extensions><TPX xmlns=\"http://www.garmin.com/xmlschemas/ActivityExtension/v2\"><Watts>171</Watts></TPX></Extensions></Trackpoint><Trackpoint><Time>2008-03-03T14:04:48Z</Time><Position><LatitudeDegrees>35.861005</LatitudeDegrees><LongitudeDegrees>-78.896878</LongitudeDegrees></Position><AltitudeMeters>94.347</AltitudeMeters><DistanceMeters>8739.119</DistanceMeters><Cadence>78</Cadence><Extensions><TPX xmlns=\"http://www.garmin.com/xmlschemas/ActivityExtension/v2\"><Watts>174</Watts></TPX></Extensions></Trackpoint><Trackpoint><Time>2008-03-03T14:04:49Z</Time><Position><LatitudeDegrees>35.860983</LatitudeDegrees><LongitudeDegrees>-78.896748</LongitudeDegrees></Position><AltitudeMeters>93.866</AltitudeMeters><DistanceMeters>8751.079</DistanceMeters><Cadence>78</Cadence><Extensions><TPX xmlns=\"http://www.garmin.com/xmlschemas/ActivityExtension/v2\"><Watts>174</Watts></TPX></Extensions></Trackpoint><Trackpoint><Time>2008-03-03T14:04:50Z</Time><Position><LatitudeDegrees>35.860961</LatitudeDegrees><LongitudeDegrees>-78.896622</LongitudeDegrees></Position><AltitudeMeters>93.866</AltitudeMeters><DistanceMeters>8762.634</DistanceMeters><Cadence>75</Cadence><Extensions><TPX xmlns=\"http://www.garmin.com/xmlschemas/ActivityExtension/v2\"><Watts>151</Watts></TPX></Extensions></Trackpoint><Trackpoint><Time>2008-03-03T14:04:51Z</Time><Position><LatitudeDegrees>35.860939</LatitudeDegrees><LongitudeDegrees>-78.896498</LongitudeDegrees></Position><AltitudeMeters>93.385</AltitudeMeters><DistanceMeters>8774.146</DistanceMeters><Cadence>75</Cadence><Extensions><TPX xmlns=\"http://www.garmin.com/xmlschemas/ActivityExtension/v2\"><Watts>150</Watts></TPX></Extensions></Trackpoint><Trackpoint><Time>2008-03-03T14:04:52Z</Time><Position><LatitudeDegrees>35.860917</LatitudeDegrees><LongitudeDegrees>-78.896373</LongitudeDegrees></Position><AltitudeMeters>92.905</AltitudeMeters><DistanceMeters>8785.588</DistanceMeters><Cadence>78</Cadence><Extensions><TPX xmlns=\"http://www.garmin.com/xmlschemas/ActivityExtension/v2\"><Watts>141</Watts></TPX></Extensions></Trackpoint><Trackpoint><Time>2008-03-03T14:04:53Z</Time><Position><LatitudeDegrees>35.860922</LatitudeDegrees><LongitudeDegrees>-78.896254</LongitudeDegrees></Position><AltitudeMeters>92.424</AltitudeMeters><DistanceMeters>8796.207</DistanceMeters><Cadence>79</Cadence><Extensions><TPX xmlns=\"http://www.garmin.com/xmlschemas/ActivityExtension/v2\"><Watts>138</Watts></TPX></Extensions></Trackpoint><Trackpoint><Time>2008-03-03T14:04:54Z</Time><Position><LatitudeDegrees>35.860921</LatitudeDegrees><LongitudeDegrees>-78.896131</LongitudeDegrees></Position><AltitudeMeters>91.943</AltitudeMeters><DistanceMeters>8807.316</DistanceMeters><Cadence>81</Cadence><Extensions><TPX xmlns=\"http://www.garmin.com/xmlschemas/ActivityExtension/v2\"><Watts>112</Watts></TPX></Extensions></Trackpoint><Trackpoint><Time>2008-03-03T14:04:55Z</Time><Position><LatitudeDegrees>35.860919</LatitudeDegrees><LongitudeDegrees>-78.896003</LongitudeDegrees></Position><AltitudeMeters>91.463</AltitudeMeters><DistanceMeters>8818.834</DistanceMeters><Cadence>82</Cadence><Extensions><TPX xmlns=\"http://www.garmin.com/xmlschemas/ActivityExtension/v2\"><Watts>106</Watts></TPX></Extensions></Trackpoint><Trackpoint><Time>2008-03-03T14:04:56Z</Time><Position><LatitudeDegrees>35.860918</LatitudeDegrees><LongitudeDegrees>-78.895874</LongitudeDegrees></Position><AltitudeMeters>90.982</AltitudeMeters><DistanceMeters>8830.497</DistanceMeters><Cadence>82</Cadence><Extensions><TPX 
